vi "Sawtooth generation VI.vi"(0 "physical channels":tag="Dev2/ao1", 1 "Sawtooth generator":T1={"Amplitude [V]"=1.0, "Offset [V]"=0.0, "Frequency (Hz)"=50.0} {"Frequency (Hz)" min=-50.0 max=50.0 step=0.00010000000000000003 format="%#_13g"; "Offset [V]" format="%.2p"; "Amplitude [V]" min=-0.7 max=0.7 format="%.2p"}) -> (7 "Waveform Graph":waveform(dbl)(graph))   [LabVIEW 2020]
uses:
  typedefs/typedef_sawtooth_control.ctl
  <vilib>/DAQmx/write.llb/DAQmx Write (Analog Wfm 1Chan NSamp).vi
  <vilib>/DAQmx/create/channels.llb/DAQmx Create Channel (AO-Voltage-Basic).vi
  Global stop DAQ.vi
  <vilib>/DAQmx/configure/timing.llb/DAQmx Timing (Sample Clock).vi
  <vilib>/DAQmx/miscellaneous.llb/DAQmx Fill In Error Info.vi
  <vilib>/measure/NI_MABase.lvlib
panel:
  out "number of samples written per channel":u32
  in  "stop":bool
  # "Fs= sampling rate in samples per second\n#s= number of samples in the waveform"
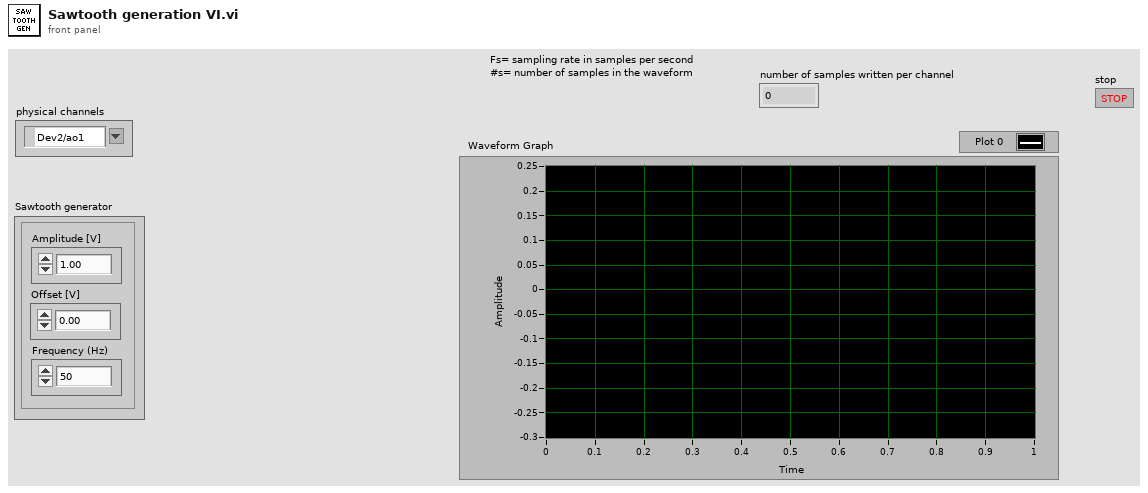
[diagram p1: front panel]
types:
  T1 = typedef "typedef_sawtooth_control.ctl" = cluster{"Amplitude [V]":dbl, "Offset [V]":dbl, "Frequency (Hz)":dbl}
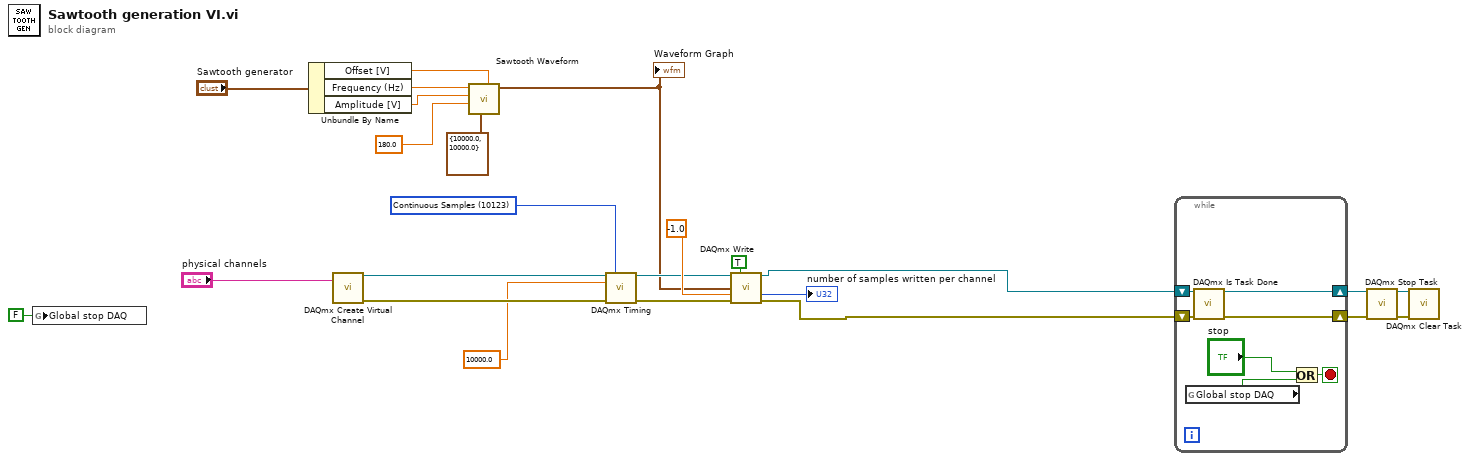
[diagram p0: block diagram]
diagram:
  w20 = 10123 items=["Finite Samples"=10178, "Continuous Samples"=10123, "Hardware Timed Single Point"=12522] ("sample mode")
  n1 = global write "Global stop DAQ.vi" "Global stop DAQ"(FALSE ("Global stop DAQ")) -> ()
  n2 = Unbundle By Name("Sawtooth generator") -> ("Offset [V]"=w8:dbl, "Frequency (Hz)"=w1:dbl, "Amplitude [V]"=w7:dbl)
  n3 = call-poly <vilib>:"DAQmx Create Virtual Channel.vi"("physical channels"="physical channels") -> ("task out"=w22:refnum<k21>, "error out"=w21:errorcluster)  [unwired: 13 in]
  n4 = call <vilib>:"Sawtooth Waveform.vi"("offset"=w8, "sampling info"=cluster{"Fs":dbl, "#s":dbl} {"Fs"=10000.0, "#s"=10000.0}, "phase"=180.0 ("y"), "amplitude"=w7, "frequency"=w1) -> ("signal out"=w10:waveform(dbl))  [unwired: 5 in, 1 out]
  "Waveform Graph" <- w10
  n5 = call-poly <vilib>:"DAQmx Timing.vi"("task/channels in"=w22, "sample mode"=w20, "rate"=10000.0, "error in"=w21) -> ("task out"=w16:refnum<k21>, "error out"=w15:errorcluster)  [unwired: 10 in]
  n6 = call-poly <vilib>:"DAQmx Write.vi"("task/channels in"=w16, "auto start"=TRUE, "data"=w10, "timeout"=-1.0, "error in"=w15) -> ("task out"=w18:refnum<k21>, "number of samples written per channel"=→"number of samples written per channel":u32, "error out"=w19:errorcluster)  [unwired: 8 in]
  n7 = while {
    shift-right: [w28] -> w13
    shift-left: w18 -> [w31]
    shift-right: [w29] -> w14
    shift-left: w19 -> [w30]
    stop <- w27 stop-if-true
    n8 = global read "Global stop DAQ.vi" "Global stop DAQ"() -> (w26:bool)
    n9 = call <vilib>:"DAQmx Is Task Done.vi"("task/channels in"=w31, "error in"=w30) -> ("task out"=w28:refnum<k21>, "error out"=w29:errorcluster)  [unwired: 11 in, 1 out]
    n10 = Or(x="stop", y=w26) -> (x .or. y?=w27:bool)
  }
  n11 = call <vilib>:"DAQmx Stop Task.vi"("task/channels in"=w13, "error in"=w14) -> ("task out"=w23:refnum<k21>, "error out"=w24:errorcluster)  [unwired: 12 in]
  n12 = call <vilib>:"DAQmx Clear Task.vi"("task in"=w23, "error in"=w24) -> ()  [unwired: 13 in, 1 out]
